vi "Add VI.vi"(6 "only accept open windows? (F)":bool, 8 "error in":errorcluster, 9 "VIs to exclude":variant, 10 "VI ref":refnum<vi>, 11 "state in":T1) -> (0 "error out":errorcluster, 3 "state out":T1)   [LabVIEW 2010, in "NI_SE_Config Front Panel Layout.lvlib"]
uses:
  NI_SE_Config Front Panel Layout.lvlib
  State.ctl
  VI Info.ctl
  VI Panel Layout/VI Panel Layout.lvclass
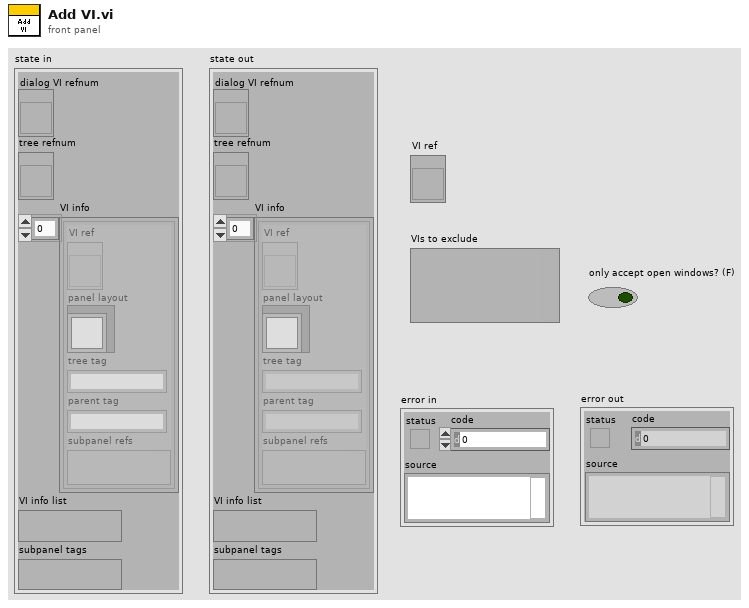
[diagram p1: front panel]
types:
  T1 = typedef "NI_SE_Config Front Panel Layout.lvlib/State.ctl" = cluster{"dialog VI refnum":refnum<vi>, "tree refnum":refnum<vi>, "VI info":T2[], "VI info list":variant, "subpanel tags":variant}
  T2 = typedef "NI_SE_Config Front Panel Layout.lvlib/VI Info.ctl" = cluster{"VI ref":refnum<vi>, "panel layout":refnum<class "VI Panel Layout.lvclass">, "tree tag":string, "parent tag":string, "subpanel refs":variant}
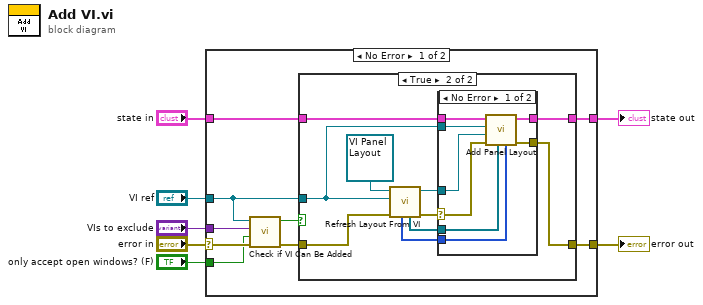
[diagram p0: block diagram]
diagram:
  n1 = case shown="No Error" "error in" {
    selector: "error in" -> [w12 w39]
    tunnel: "state in" -> [w16 w40]
    tunnel: [w15 w40] -> w5
    tunnel: [w14 w39] -> w4
    tunnel: "VI ref" -> [w13 _]
    tunnel: "VIs to exclude" -> [w10 _]
    tunnel: "only accept open windows? (F)" -> [w8 _]
    frame No Error {
      n2 = call "Check if VI Can Be Added.vi"("error in"=w12, "only accept open windows? (F)"=w8, "VIs to exclude"=w10, "VI refnum"=w13) -> ("error out"=w11:errorcluster, "allowed?"=w9:bool)  [unwired: 6 in]
      n3 = case shown="True" w9 {
        tunnel: w16 -> [w17 w28]
        tunnel: [w17 w27] -> w15
        tunnel: [w18 w26] -> w14
        tunnel: w13 -> [_ w24]
        tunnel: w11 -> [w18 w22]
        frame False {
        }
        frame True {
          n4 = call "Refresh Layout From VI.vi"("error in (no error)"=w22, "VI refnum"=w24, "VI Panel Layout in"=refnum<class "VI Panel Layout.lvclass"> refnum ("VI Panel Layout out")) -> ("error out"=w19:errorcluster, "VI Panel Layout out"=w23:refnum<class "VI Panel Layout.lvclass">, "subpanel refnums"=w21:refnum<vi>[], "subpanel UIDs"=w20:i32[])  [unwired: 5 in]
          n5 = case shown="No Error" w19 {
            selector: w19 -> [w29 w37]
            tunnel: w28 -> [w36 w38]
            tunnel: [w35 w38] -> w27
            tunnel: [w34 w37] -> w26
            tunnel: w24 -> [w33 _]
            tunnel: w23 -> [w32 _]
            tunnel: w21 -> [w31 _]
            tunnel: w20 -> [w30 _]
            frame No Error {
              n6 = call "Add Panel Layout.vi"("subpanel UIDs"=w30, "subpanel refnums"=w31, "error in"=w29, "panel layout"=w32, "VI ref"=w33, "state in"=w36) -> ("error out"=w34:errorcluster, "state out"=w35:T1)  [unwired: 3 in, 1 out]
            }
            frame Error {
            }
          }
        }
      }
    }
    frame Error {
    }
  }
  "state out" <- w5
  "error out" <- w4
